vi "XOR chksum.vi"(1 "String":string="hello") -> (0 "Checksum":string)   [LabVIEW 2016]
panel:
  # "Performs bitwise xor on each byte in input string."
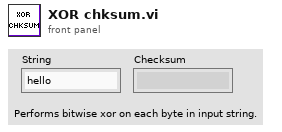
[diagram p1: front panel]
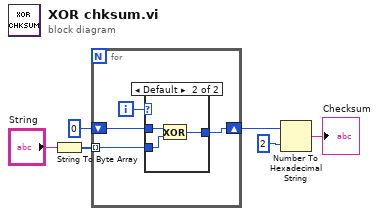
[diagram p0: block diagram]
diagram:
  n1 = String To Byte Array(string="String") -> (unsigned byte array=w5:u8[])
  n2 = for {
    tunnel: w5 -> [w9] mode=indexing
    shift-right: [w7] -> w3
    shift-left: u8 0 -> [w8]
    i -> [w10]
    n3 = case shown="Default" w10 {
      tunnel: [w11 w12] -> w7
      tunnel: w9 -> [w11 w13]
      tunnel: w8 -> [_ w14]
      frame 0 {
      }
      frame Default {
        n4 = Exclusive Or(1:w13, 2:w14) -> (0:w12:u8)
      }
    }
  }
  n5 = Number To Hexadecimal String(1:i16 2 ("width (-)"), 2:w3) -> (0:→"Checksum":string)
